vi "BuildAction.vi"() -> (1 "Path":path, 2 "VI Path":path, 3 "Application Directory":path)   [LabVIEW 2020, in "epl-network.lvlib"]
uses:
  epl-network.lvlib
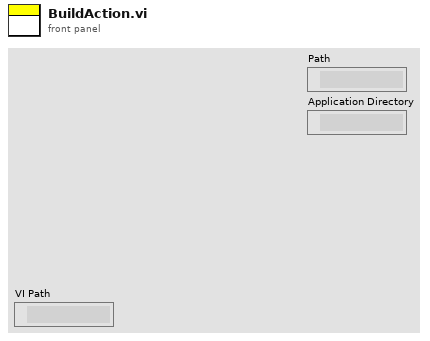
[diagram p1: front panel]
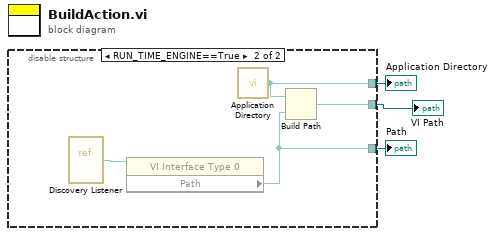
[diagram p0: block diagram]
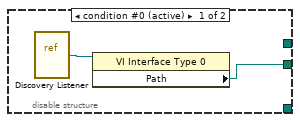
[diagram p2: hidden frame]
diagram:
  n1 = disable-structure shown="RUN_TIME_ENGINE==True" {
    disable-tunnel: [w4 w9] -> w3
    disable-tunnel: [_ w7] -> w2
    disable-tunnel: [_ w6] -> w1
    frame condition #0 (active) {
      n2 = vi-ref "Discovery Listener.vi"() -> (w5:refnum<vi>)
      n3 = property class="VI Interface Type 0"(reference=w5) -> ("Path"=w4:path)  [unwired: 1 in, 2 out]
    }
    frame condition #1 {
      n4 = vi-ref "Discovery Listener.vi"() -> (w8:refnum<vi>)
      n5 = property class="VI Interface Type 0"(reference=w8) -> ("Path"=w7:path)  [unwired: 1 in, 2 out]
      n6 = call <vilib>:"Application Directory.vi"() -> ("Application Directory"=w6:path)
      n7 = Build Path(base path=w6, name or relative path=w7) -> (appended path=w9:path)
    }
  }
  "VI Path" <- w3
  "Path" <- w2
  "Application Directory" <- w1
